vi "AlliGator Python Plugin Function Doc String.vi"(8 "Error In":errorcluster, 9 "Source":string, 11 "String in":string) -> (0 "Error Out":errorcluster, 1 "Doc String":string, 3 "String out":string)   [LabVIEW 2021, in "AlliGator Python Plugins.lvlib"]
doc: "Extracts doc string from python function."
uses:
  AlliGator Python Plugins.lvlib
  Strings/Strings.lvlib
panel:
  # "see the AlliGator License on the block diagram (Ctrl+E or Window:Show Block Diagram)"
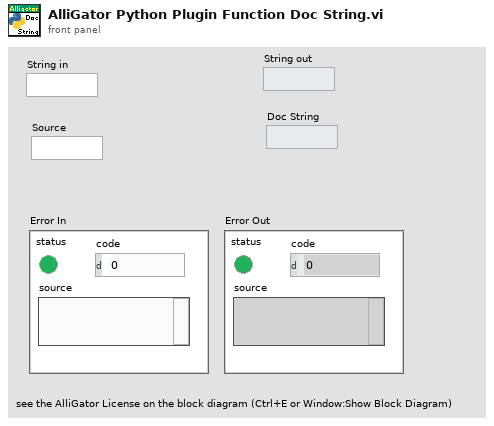
[diagram p1: front panel]
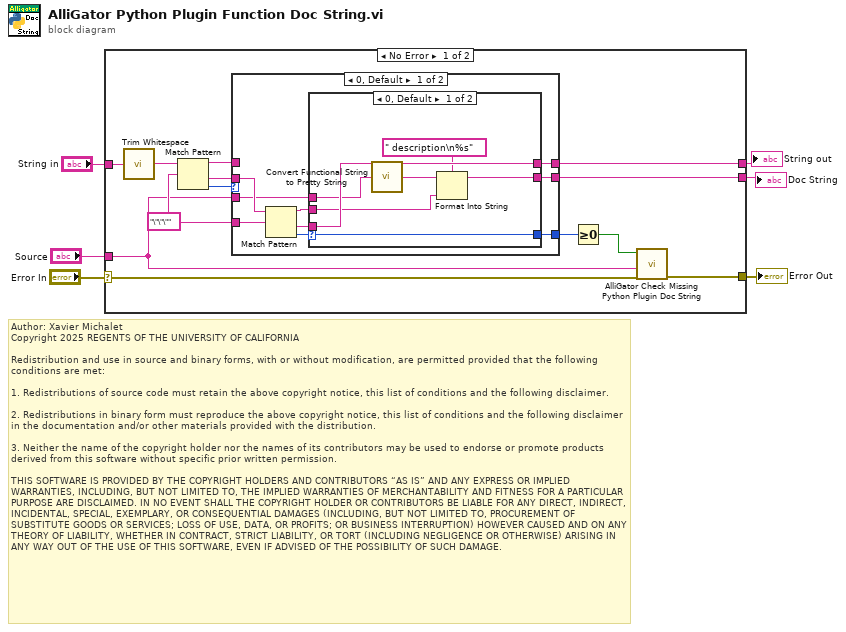
[diagram p0: block diagram]
diagram:
  # "Author: Xavier Michalet\nCopyright 2025 REGENTS OF THE UNIVERSITY OF CALIFORNIA\n\nRedistribution and use in source and binary forms, with or without modification, are permitted provided that the following conditions are met:\n\n1. Redistributions of source code must retain the above copyright notice, this list of conditions and the following disclaimer.\n\n2. Redistributions in binary form must reproduce the above copyright notice, this list of conditions and the following disclaimer in the documentation and/or other materials provided with the distribution.\n\n3. Neither the name of the copyright holder nor the names of its contributors may be used to endorse or promote products derived from this software without specific prior written permission.\n\nTHIS SOFTWARE IS PROVIDED BY THE COPYRIGHT HOLDERS AND CONTRIBUTORS “AS IS” AND ANY EXPRESS OR IMPLIED WARRANTIES, INCLUDING, BUT NOT LIMITED TO, THE IMPLIED WARRANTIES OF MERCHANTABILITY AND FITNESS FOR A PARTICULAR PURPOSE ARE DISCLAIMED. IN NO EVENT SHALL THE COPYRIGHT HOLDER OR CONTRIBUTORS BE LIABLE FOR ANY DIRECT, INDIRECT, INCIDENTAL, SPECIAL, EXEMPLARY, OR CONSEQUENTIAL DAMAGES (INCLUDING, BUT NOT LIMITED TO, PROCUREMENT OF SUBSTITUTE GOODS OR SERVICES; LOSS OF USE, DATA, OR PROFITS; OR BUSINESS INTERRUPTION) HOWEVER CAUSED AND ON ANY THEORY OF LIABILITY, WHETHER IN CONTRACT, STRICT LIABILITY, OR TORT (INCLUDING NEGLIGENCE OR OTHERWISE) ARISING IN ANY WAY OUT OF THE USE OF THIS SOFTWARE, EVEN IF ADVISED OF THE POSSIBILITY OF SUCH DAMAGE."
  n1 = case shown="No Error" "Error In" {
    selector: "Error In" -> [w9 w40]
    tunnel: "String in" -> [w19 w41]
    tunnel: [w18 w41] -> w5
    tunnel: [w17 _] -> w4
    tunnel: [w8 w40] -> w2
    tunnel: "Source" -> [w7 _]
    frame No Error {
      w16 = "\"\"\"" ("regular expression")
      n2 = call <vilib>:"Trim Whitespace.vi"("string"=w19) -> ("trimmed string"=w14:string)  [unwired: 1 in]
      n3 = Match Pattern(string=w14, regular expression=w16) -> (before substring=w12:string, after substring=w15:string, offset past match=w13:i32)  [unwired: 1 in, 1 out]
      n4 = case shown="0, Default" w13 {
        selector: w13 -> [_ w38]
        tunnel: [w23 w39] -> w18
        tunnel: [w24 _] -> w17
        tunnel: w16 -> [w28 _]
        tunnel: w15 -> [w27 _]
        tunnel: w12 -> [_ w39]
        tunnel: [w21 w38] -> w11
        tunnel: w7 -> [w20 _]
        frame 0, Default {
          n5 = Match Pattern(string=w27, regular expression=w28) -> (before substring=w25:string, after substring=w22:string, offset past match=w26:i32)  [unwired: 1 in, 1 out]
          n6 = case shown="0, Default" w26 {
            selector: w26 -> [w34 w36]
            tunnel: w25 -> [w32 w37]
            tunnel: [w33 _] -> w24
            tunnel: [w35 w37] -> w23
            tunnel: w22 -> [w35 _]
            tunnel: [w34 w36] -> w21
            tunnel: w20 -> [w31 _]
            frame 0, Default {
              n7 = call "Convert Functional String to Pretty String.vi"("Functional Name"=w31) -> ("Pretty Name"=w29:string)  [unwired: 4 in]
              n8 = Format Into String(format string=" description\n%s", initial string=w29, w32) -> (resulting string=w33:string)  [unwired: 1 in, 1 out]
            }
            frame -1 {
            }
          }
        }
        frame -1 {
        }
      }
      n9 = Greater Or Equal To 0?(x=w11) -> (x >= 0?=w10:bool)
      n10 = call "AlliGator Check Missing Python Plugin Doc String.vi"("error in (no error)"=w9, "Source"=w7, "Doc String Found"=w10) -> ("error out"=w8:errorcluster)  [unwired: 8 in]
    }
    frame Error {
    }
  }
  "String out" <- w5
  "Doc String" <- w4
  "Error Out" <- w2
